vi "FTW-Request-AddExceptionToResponse.vi"(0 "Response":refnum<data-value>, 11 "error in":errorcluster) -> (4 "Response out":refnum<data-value>, 15 "error out":errorcluster)   [LabVIEW 2014]
doc: "Sends a response message back to the requesting client. This message is attempts to send unconditionally of incoming error. Take caution to wire a sanitized error into this function, because it will be repeated back onto the client. Said another way, an error generated while processing the request will be not only thrown on the request handler, but also on the client as well."
uses:
  json/core/FTW-JSON-Core-Structure.ctl
panel:
  # "Inputs"
  # "Outputs"
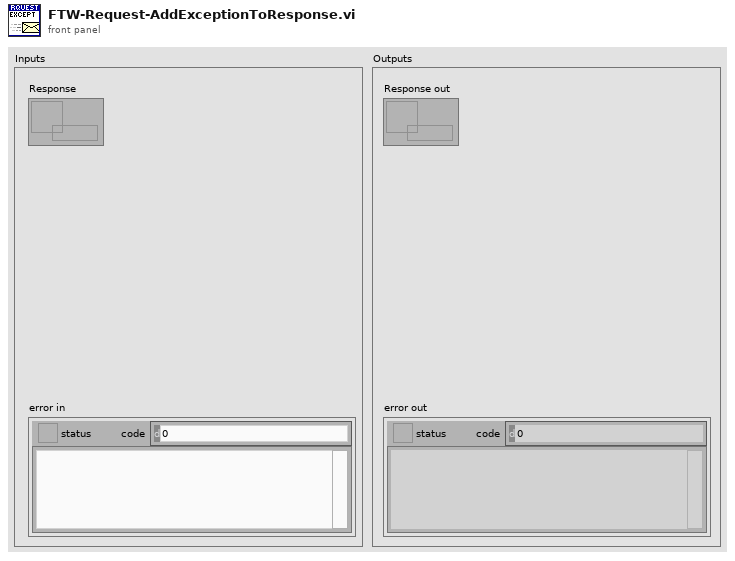
[diagram p1: front panel]
types:
  T1 = typedef "FTW-ERR-ExceptionType.ctl" = enum16{"OK", "Info", "Warning", "Error"}
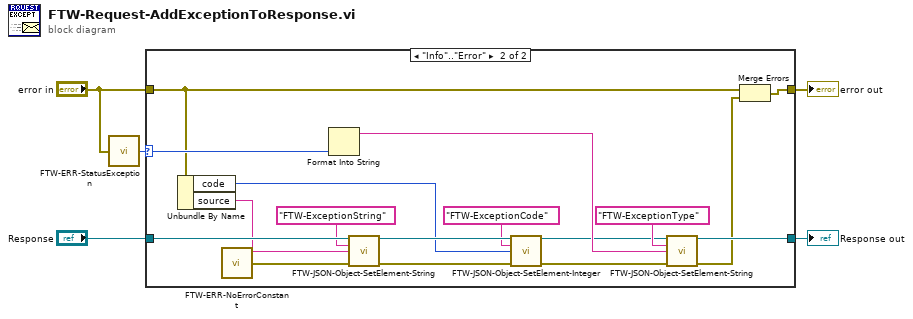
[diagram p0: block diagram]
diagram:
  n1 = call "FTW-ERR-StatusException.vi"("error to check"="error in") -> ("Exception"=w5:T1)
  n2 = case shown="\"Info\"..\"Error\"" w5 {
    selector: w5 -> [_ w22]
    tunnel: "Response" -> [w7 w24]
    tunnel: [w7 w21] -> w2
    tunnel: "error in" -> [w6 w9]
    tunnel: [w6 w11] -> w1
    frame "OK" {
    }
    frame "Info".."Error" {
      n3 = Unbundle By Name(w9) -> ("code"=w16:i32, "source"=w14:string)
      n4 = call "FTW-ERR-NoErrorConstant.vi"() -> ("no error"=w8:errorcluster)
      n5 = Format Into String(w22) -> (resulting string=w19:string)  [unwired: 3 in, 1 out]
      n6 = call "FTW-JSON-Object-SetElement-String.vi"("JSON Object"=w24, "Key"="FTW-ExceptionString", "Value"=w14, "error in"=w8) -> ("JSON Object out"=w18:refnum<data-value>, "error out"=w13:errorcluster)  [unwired: 10 in]
      n7 = call "FTW-JSON-Object-SetElement-Integer.vi"("JSON Object"=w18, "Key"="FTW-ExceptionCode", "Value"=w16, "error in"=w13) -> ("JSON Object out"=w17:refnum<data-value>, "error out"=w12:errorcluster)  [unwired: 10 in]
      n8 = call "FTW-JSON-Object-SetElement-String.vi"("JSON Object"=w17, "Key"="FTW-ExceptionType", "Value"=w19, "error in"=w12) -> ("JSON Object out"=w21:refnum<data-value>, "error out"=w10:errorcluster)  [unwired: 10 in]
      n9 = Merge Errors(w9, w10) -> (w11:errorcluster)
    }
  }
  "error out" <- w1
  "Response out" <- w2
